vi "Implement Dynamic Dispatch VIs.vi"(8 "error in (no error)":errorcluster, 11 "Mock Class Generator In":refnum<class "Pure Mock Class Generator.lvclass">) -> (0 "error out":errorcluster, 3 "Mock Class Generator Out":refnum<class "Pure Mock Class Generator.lvclass">)   [LabVIEW 2020, in "Pure Mock Class Generator.lvclass"]
uses:
  Pure Mock Class Generator.lvclass
  Pure Mock Class Generator.lvclass/Pure Mock Class Generator.ctl
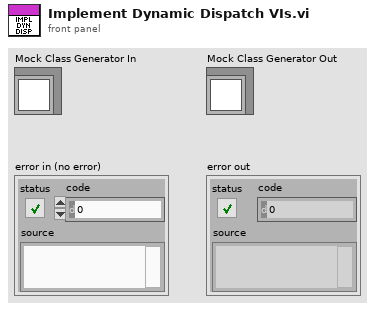
[diagram p1: front panel]
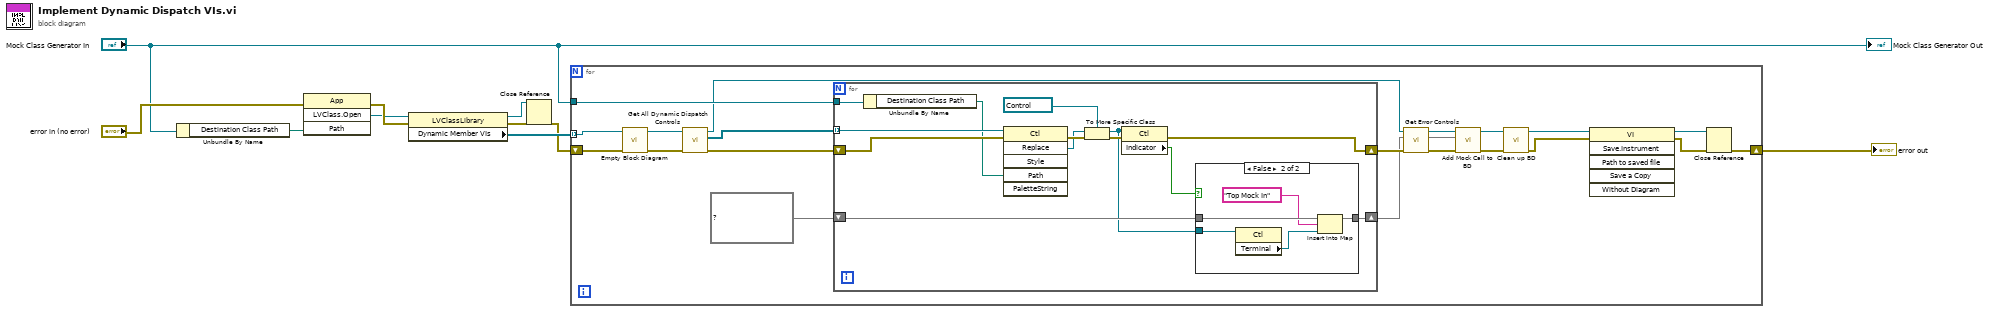
[diagram p0: block diagram]
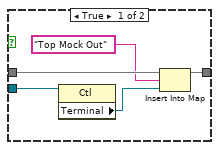
[diagram p2: hidden frame]
diagram:
  n1 = Unbundle By Name("Mock Class Generator In") -> ("Destination Class Path"=w10:path)
  n2 = invoke class="App" method="LVClass.Open"(error in="error in (no error)", "Path"=w10) -> (error out=w9:errorcluster, "LVClass.Open"=w4:refnum<vi>)  [unwired: 2 in, 2 out]
  n3 = property class="LVClassLibrary"(reference=w4, error in=w9) -> (reference out=w5:refnum<vi>, error out=w6:errorcluster, "Dynamic Member VIs"=w7:refnum<vi>[])
  n4 = Close Reference(reference=w5, error in (no error)=w6) -> (error out=w3:errorcluster)
  n5 = for {
    tunnel: w7 -> [w16] mode=indexing
    tunnel: "Mock Class Generator In" -> [w30]
    shift-right: [w28] -> w1
    shift-left: w3 -> [w12]
    n6 = call "Empty Block Diagram.vi"("error in (no error)"=w12, "VI in"=w16) -> ("error out"=w13:errorcluster, "reference out"=w27:refnum<vi>)  [unwired: 8 in]
    n7 = call "Get All Dynamic Dispatch Controls.vi"("error in (no error)"=w13, "VI in"=w27) -> ("error out"=w31:errorcluster, "Dynamic Dispatch Controls"=w29:refnum<vi>[], "reference out"=w25:refnum<vi>)  [unwired: 7 in]
    n8 = for {
      tunnel: w29 -> [w44] mode=indexing
      shift-right: [w36] -> w26
      shift-left: w31 -> [w43]
      tunnel: w30 -> [w42]
      shift-right: [w34] -> w21
      shift-left: map{string, refnum<vi>} {} ("map") -> [w35]
      n9 = Unbundle By Name(w42) -> ("Destination Class Path"=w41:path)
      n10 = invoke class="Ctl" method="Replace"(reference=w44, error in=w43, "Path"=w41) -> (error out=w40:errorcluster, "Replace"=w38:refnum<vi>)  [unwired: 3 in, 4 out]
      n11 = To More Specific Class(target class=refnum<vi> refnum ("reference out"), reference=w38, error in=w40) -> (specific class reference=w32:refnum<vi>, error out=w39:errorcluster)
      n12 = property class="Ctl"(reference=w32, error in=w39) -> (error out=w36:errorcluster, "Indicator"=w33:bool)  [unwired: 1 out]
      n13 = case shown="False" w33 {
        tunnel: w35 -> [w49 w54]
        tunnel: [w48 w53] -> w34
        tunnel: w32 -> [w46 w51]
        frame True {
          n14 = property class="Ctl"(reference=w46) -> ("Terminal"=w45:refnum<vi>)  [unwired: 1 in, 2 out]
          n15 = Insert Into Map(map in=w49, key="Top Mock Out", value=w45) -> (map out=w48:map{string, refnum<vi>})  [unwired: 2 out]
        }
        frame False {
          n16 = property class="Ctl"(reference=w51) -> ("Terminal"=w50:refnum<vi>)  [unwired: 1 in, 2 out]
          n17 = Insert Into Map(map in=w54, key="Top Mock In", value=w50) -> (map out=w53:map{string, refnum<vi>})  [unwired: 2 out]
        }
      }
    }
    n18 = call "Get Error Controls.vi"("error in (no error)"=w26, "map"=w21, "VI in"=w25) -> ("error out"=w23:errorcluster, "map out"=w20:map{string, refnum<vi>}, "reference out"=w24:refnum<vi>)  [unwired: 6 in]
    n19 = call "Add Mock Call to BD.vi"("error in (no error)"=w23, "map"=w20, "VI in"=w24) -> ("error out"=w14:errorcluster, "VI out"=w19:refnum<vi>)  [unwired: 7 in]
    n20 = call "Clean up BD.vi"("error in (no error)"=w14, "VI in"=w19) -> ("error out"=w15:errorcluster, "VI out"=w18:refnum<vi>)  [unwired: 8 in]
    n21 = invoke class="VI" method="Save.Instrument"(reference=w18, error in=w15) -> (reference out=w17:refnum<vi>, error out=w11:errorcluster)  [unwired: 4 in, 4 out]
    n22 = Close Reference(reference=w17, error in (no error)=w11) -> (error out=w28:errorcluster)
  }
  "error out" <- w1
  "Mock Class Generator Out" <- "Mock Class Generator In"
